vi "Sample Out.vi"(8 "error in (no error)":errorcluster, 11 "Syringe in":refnum<class "Syringe Line.lvclass">) -> (0 "error out":errorcluster, 3 "Syringe out":refnum<class "Syringe Line.lvclass">)   [LabVIEW 2015, in "cRIO-Carbondioxide.lvlib" / "CO2-Actor.lvlib" / "Syringe Line.lvclass"]
uses:
  Syringe Line.lvclass
  CO2 Actor/CO2 Actor.lvclass
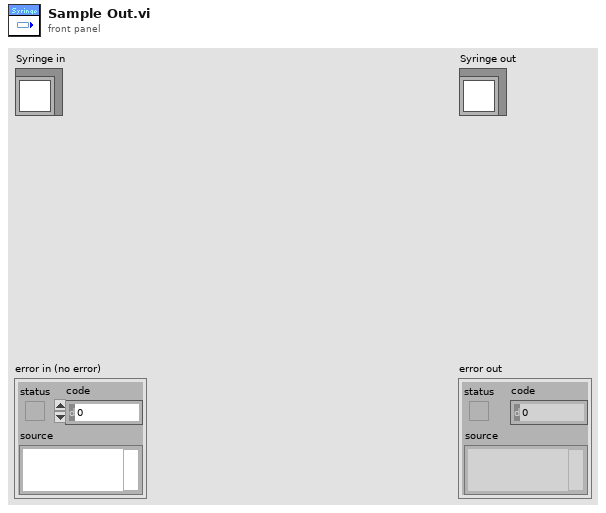
[diagram p1: front panel]
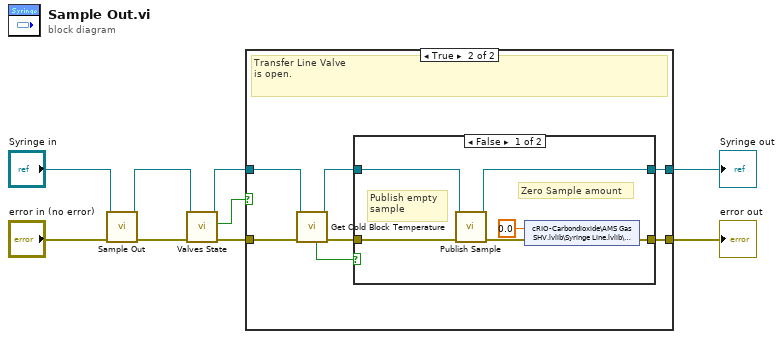
[diagram p0: block diagram]
diagram:
  n1 = call-parent "Sample Out.vi"("error in (no error)"="error in (no error)", "CO2 Actor in"="Syringe in") -> ("error out"=w7:errorcluster, "CO2 Actor out"=w6:refnum<class "Syringe Line.lvclass">)  [unwired: 8 in]
  n2 = call "Valves State.vi"("error in (no error)"=w7, "Syringe in"=w6) -> ("error out"=w4:errorcluster, "Valve Transfer Line Open"=w1:bool, "Syringe out"=w3:refnum<class "Syringe Line.lvclass">)  [unwired: 6 in, 1 out]
  n3 = case shown="True" w1 {
    tunnel: [w10 w18] -> w5
    tunnel: w4 -> [w10 w16]
    tunnel: w3 -> [w11 w14]
    tunnel: [w11 w17] -> w2
    frame False {
    }
    frame True {
      # "Transfer Line Valve\nis open."
      n4 = call "Get Cold Block Temperature.vi"("error in (no error)"=w16, "Syringe Line in"=w14) -> ("error out"=w15:errorcluster, "Syringe Line out"=w13:refnum<class "Syringe Line.lvclass">, "Frozen?"=w12:bool)  [unwired: 6 in, 1 out]
      n5 = case shown="False" w12 {
        tunnel: [w20 w25] -> w18
        tunnel: [w24 w26] -> w17
        tunnel: w15 -> [w22 w25]
        tunnel: w13 -> [w23 w26]
        frame False {
          # "Zero Sample amount"
          # "Publish empty\nsample"
          n6 = call "Publish Sample.vi"("error in (no error)"=w22, "Syringe Line in"=w23) -> ("error out"=w21:errorcluster, "Syringe Line out"=w24:refnum<class "Syringe Line.lvclass">)  [unwired: 8 in]
          n7 = shared-variable "cRIO-Carbondioxide\\AMS Gas SHV.lvlib\\Syringe Line.lvlib\\Sample mBar"(0.0 ("Sample mBar"), error in=w21) -> (error out=w20:errorcluster)
        }
        frame True {
        }
      }
    }
  }
  "error out" <- w5
  "Syringe out" <- w2
